vi "Async Initialize.vi"(8 "error in (no error)":errorcluster, 10 "RT Configuration":T1 {"Frames"."Protection Configurations"."CRC Channels"."Data Type" items=["Signed", "Unsigned", "IEEE Float"]}, 11 "Process in":refnum<class "Process.lvclass">) -> (0 "error out":errorcluster, 2 "Execute":bool, 3 "Variables":T9)   [LabVIEW 2019, in "Protection and Counter Addon Engine.lvlib"]
uses:
  Protection and Counter Addon Engine.lvlib
  Types/RT Async Engine Variables.ctl
  <vilib>/NI/NIVS Inline Async API/_VS Inline Async API/Process/Process.lvclass
  <vilib>/NI/NI VeriStand Addon Network Comm/Engine/VeriStand Comm.lvclass
  Types/RT Data References.ctl
  <vilib>/NI/NIVS Inline Async API/_Data Access Engine/Data Access Engine/Types/Write.DVR.ctl
  <vilib>/NI/NIVS Inline Async API/_Data Access Engine/Access Type Classes/Write/Write.lvclass
  <vilib>/NI/NIVS Inline Async API/_Data Access Engine/Data Access Engine/Types/Read.DVR.ctl
  <vilib>/NI/NIVS Inline Async API/_Data Access Engine/Access Type Classes/Read/Read.lvclass
  Types/RT Async Engine Settings.ctl
  SubModules/Frame Protection Support/Source/Engine/Types/RT Frame Settings.ctl
  SubModules/Frame Protection Support/Source/Shared/Types/Exported Frame Type.ctl
  SubModules/Frame Protection Support/Source/Engine/Types/RT Protection Configuration.ctl
  SubModules/Frame Protection Support/Source/Shared/Types/Protection Type.ctl
  SubModules/Frame Protection Support/Source/Shared/Types/XNET Signal Configuration.ctl
  SubModules/Frame Protection Support/Source/Shared/Types/Exported Counter Settings.ctl
  SubModules/Frame Protection Support/Source/Shared/Types/Exported Event Trigger Type.ctl
  <vilib>/NI/NI VeriStand Addon Network Comm/Engine/VeriStand Comm.lvclass/VeriStand Comm.ctl
  <vilib>/NI/NIVS Inline Async API/_VS Inline Async API/Process/Process.lvclass/Process.ctl
  <vilib>/NI/NIVS Inline Async API/_VS Inline Async API/Process/Data Member Access/Read Data Access.vi
  <vilib>/NI/NIVS Inline Async API/_VS Inline Async API/Error Handling Process/SubVIs/Error.ConvertArray.vi
  Shared/SubVIs/GUID Lookup.vi
  <vilib>/Utility/SystemLogging/Write to System Log.vi
  <vilib>/NI/AMC/Create Message Queue.vi
  <vilib>/NI/STM/Connection Manager/TCP/Advanced/TCP Initialize Connection Manager (By Reference).vi
  <vilib>/NI/NIVS Inline Async API/_Data Access Engine/Data Access Engine/Methods/Read.Lookup.vi
  <vilib>/NI/NIVS Inline Async API/_Data Access Engine/Data Access Engine/Methods/Write.Lookup.vi
  <vilib>/NI/NIVS Inline Async API/_Data Access Engine/Data Access Engine/Data Access Engine.lvclass
  Shared/Protection and Counter Addon Shared.lvlib
  SubModules/Frame Protection Support/Source/Shared/Protection and Counter Support Shared.lvlib
  SubModules/Frame Protection Support/Source/Engine/Protection and Counter Support Engine.lvlib
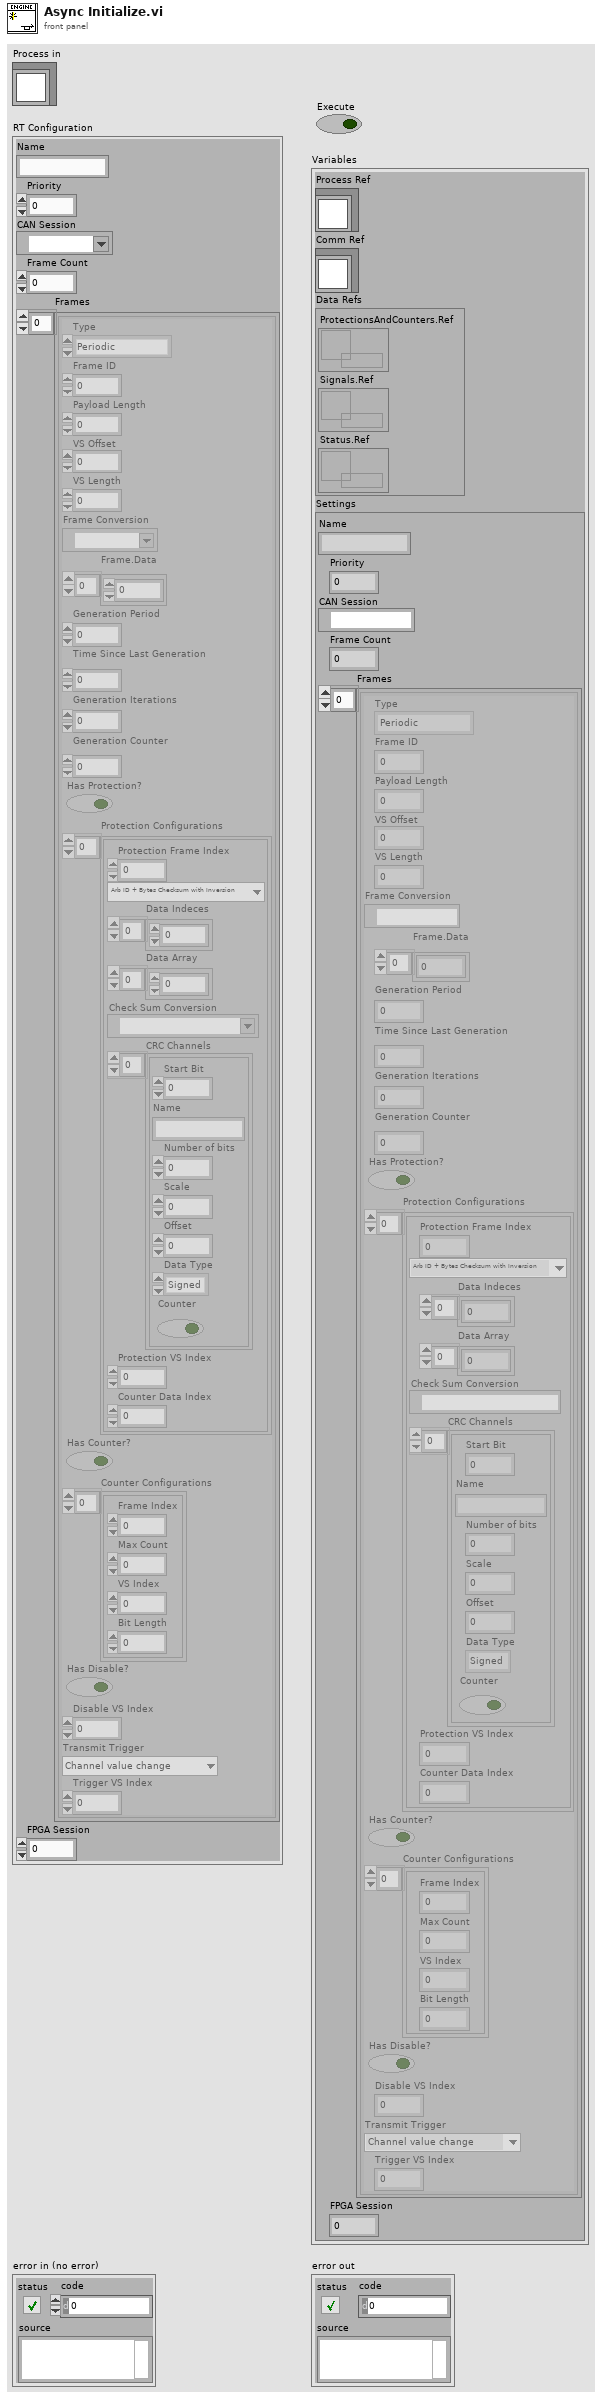
[diagram p1: front panel]
types:
  T1 = typedef "Protection and Counter Addon Engine.lvlib/RT Async Engine Settings.ctl" = cluster{"Name":string, "Priority":i32, "CAN Session":refnum<k21>, "Frame Count":i32, "Frames":T2[], "FPGA Session":u32}
  T2 = typedef "Protection and Counter Support Engine.lvlib/RT Frame Settings.ctl" = cluster{"Type":T3, "Frame ID":u32, "Payload Length":u32, "VS Offset":i32, "VS Length":i32, "Frame Conversion":refnum<k21>, "Frame.Data":dbl[], "Generation Period":u32, "Time Since Last Generation":u32, "Generation Iterations":u32, "Generation Counter":u32, "Has Protection?":bool, "Protection Configurations":T4[], "Has Counter?":bool, "Counter Configurations":T7[], "Has Disable?":bool, "Disable VS Index":i32, "Transmit Trigger":T8, "Trigger VS Index":i32}
  T3 = typedef "Protection and Counter Support Shared.lvlib/Exported Frame Type.ctl" = enum16{"Periodic", "Event", "Periodic/Event"}
  T4 = typedef "Protection and Counter Support Engine.lvlib/RT Protection Configuration.ctl" = cluster{"Protection Frame Index":i32, "Protection Type":T5, "Data Indeces":i32[], "Data Array":dbl[], "Check Sum Conversion":refnum<k21>, "CRC Channels":T6[], "Protection VS Index":i32, "Counter Data Index":i32}
  T5 = typedef "Protection and Counter Support Shared.lvlib/Protection Type.ctl" = enum16{"Arb ID + Bytes Checksum with Inversion", "Arb ID + Bytes CRC with Inversion", "Reversed Raw Signal Checksum with Inversion", "Concatenated Two's Compliment"}
  T6 = typedef "Protection and Counter Support Shared.lvlib/XNET Signal Configuration.ctl" = cluster{"Start Bit":i32, "Name":string, "Number of bits":i32, "Scale":dbl, "Offset":dbl, "Data Type":u32, "Counter":bool}
  T7 = typedef "Protection and Counter Support Shared.lvlib/Exported Counter Settings.ctl" = cluster{"Frame Index":i32, "Max Count":dbl, "VS Index":i32, "Bit Length":i64}
  T8 = typedef "Protection and Counter Support Shared.lvlib/Exported Event Trigger Type.ctl" = enum16{"Channel value change", "Trigger channel (not zero)", "Channel value change or trigger channel (not zero)", "Trigger channel (any value change)", "Channel value change or trigger channel (any value change)"}
  T9 = typedef "Protection and Counter Addon Engine.lvlib/RT Async Engine Variables.ctl" = cluster{"Process Ref":refnum<class "Process.lvclass">, "Comm Ref":refnum<class "VeriStand Comm.lvclass">, "Data Refs":T10, "Settings":T1}
  T10 = typedef "Protection and Counter Addon Engine.lvlib/RT Data References.ctl" = cluster{"ProtectionsAndCounters.Ref":T11, "Signals.Ref":T12, "Status.Ref":T11}
  T11 = typedef "Data Access Engine.lvlib/Data Access Engine.lvclass/Write.DVR.ctl" = refnum<data-value>
  T12 = typedef "Data Access Engine.lvlib/Data Access Engine.lvclass/Read.DVR.ctl" = refnum<data-value>
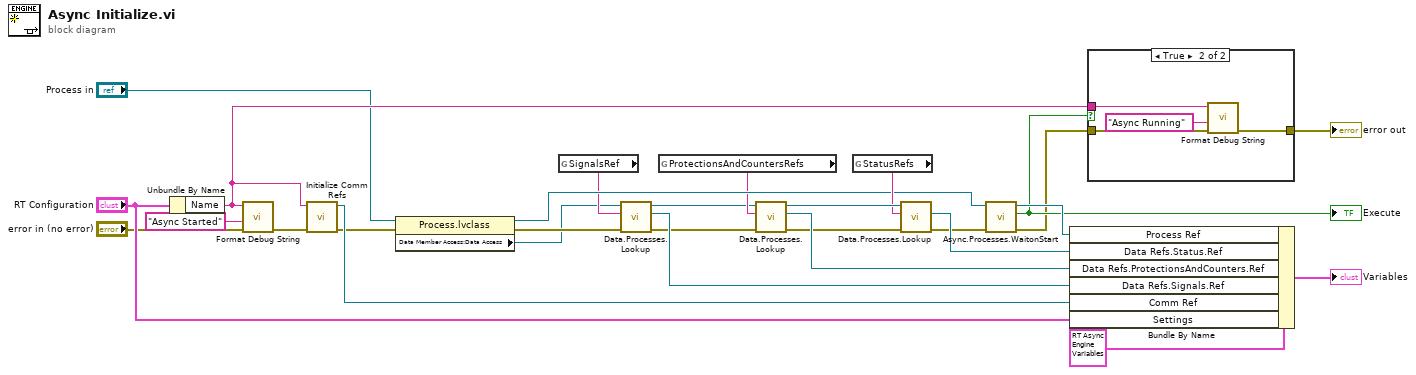
[diagram p0: block diagram]
diagram:
  n1 = Unbundle By Name("RT Configuration") -> ("Name"=w20:string)
  n2 = call "Format Debug String.vi"("error in (no error)"="error in (no error)", "State"="Async Started", "Name"=w20) -> ("error out"=w18:errorcluster)  [unwired: 8 in]
  n3 = call <vilib>:"Initialize Comm Refs.vi"("error in (no error)"=w18, "Name"=w20) -> ("error out"=w19:errorcluster, "Comm.lvclass"=w28:refnum<class "VeriStand Comm.lvclass">)  [unwired: 8 in]
  n4 = property class="Process.lvclass"(reference="Process in", error in=w19) -> (reference out=w8:refnum<class "Process.lvclass">, error out=w4:errorcluster, "Data Member Access:Data Access"=w2:refnum<class "Data Access Engine.lvclass">)
  n5 = global read "GUID Lookup.vi" "SignalsRef"() -> (w6:string)
  n6 = call-poly <vilib>:"Data.Processes.Lookup.vi"("error in (no error)"=w4, "Name"=w6, "Data Access API in"=w2) -> ("error out"=w5:errorcluster, "Ref"=w27:T12, "Data Access API out"=w3:refnum<class "Data Access Engine.lvclass">)  [unwired: 5 in, 1 out]
  n7 = global read "GUID Lookup.vi" "ProtectionsAndCountersRefs"() -> (w7:string)
  n8 = call-poly <vilib>:"Data.Processes.Lookup.vi"("error in (no error)"=w5, "Name"=w7, "Data Access API in"=w3) -> ("error out"=w11:errorcluster, "Ref"=w26:T11, "Data Access API out"=w10:refnum<class "Data Access Engine.lvclass">)  [unwired: 5 in, 1 out]
  n9 = global read "GUID Lookup.vi" "StatusRefs"() -> (w9:string)
  n10 = call-poly <vilib>:"Data.Processes.Lookup.vi"("error in (no error)"=w11, "Name"=w9, "Data Access API in"=w10) -> ("error out"=w12:errorcluster, "Ref"=w25:T11)  [unwired: 5 in, 2 out]
  n11 = call <vilib>:"Async.Processes.WaitonStart.vi"("error in (no error)"=w12, "Process"=w8) -> ("error out"=w15:errorcluster, "Execute"=w17:bool, "Process out"=w21:refnum<class "Process.lvclass">)  [unwired: 7 in]
  "Execute" <- w17
  n12 = Bundle By Name(cluster=T9 {"Process Ref"=refnum, "Comm Ref"=refnum, "Data Refs"={"ProtectionsAndCounters.Ref"=refnum, "Signals.Ref"=refnum, "Status.Ref"=refnum}, "Settings"={"Name"="", "Priority"=0, "CAN Session"="", "Frame Count"=0, "Frames"=[], "FPGA Session"=0}}, "Process Ref"=w21, "Data Refs.Status.Ref"=w25, "Data Refs.ProtectionsAndCounters.Ref"=w26, "Data Refs.Signals.Ref"=w27, "Comm Ref"=w28, "Settings"="RT Configuration") -> (→"Variables":T9)
  n13 = case shown="True" w17 {
    tunnel: w15 -> [w29 w32]
    tunnel: [w29 w31] -> w16
    tunnel: w20 -> [_ w30]
    frame False {
    }
    frame True {
      n14 = call "Format Debug String.vi"("error in (no error)"=w32, "State"="Async Running", "Name"=w30) -> ("error out"=w31:errorcluster)  [unwired: 8 in]
    }
  }
  "error out" <- w16
